vi "Load_Linnerud.vi"(8 "error in":errorcluster caption="entrée d'erreur") -> (0 "error out":errorcluster caption="sortie d'erreur", 3 "Tableau":string[][](array[string]))   [LabVIEW 2020]
doc: "Data Set Characteristics :\n\nNumber of Instances : 20\n\nNumber of Attributes : 3\n\nMissing Attribute Values : None\n\nThe Linnerud dataset is a multi-output regression dataset. It consists of three excercise (data) and three physiological (target) variables collected from twenty middle-aged men in a fitness club :\n\n - physiological - CSV containing 20 observations on 3 physiological variables : Weight, Waist and Pulse.\n\n - exercise - CSV containing 20 observations on 3 exercise variables : Chins, Situps and Jumps."
uses:
  Load_Linnerud.lvclass
panel:
  out "Load_Linnerud en sortie":refnum<class "Load_Linnerud.lvclass">
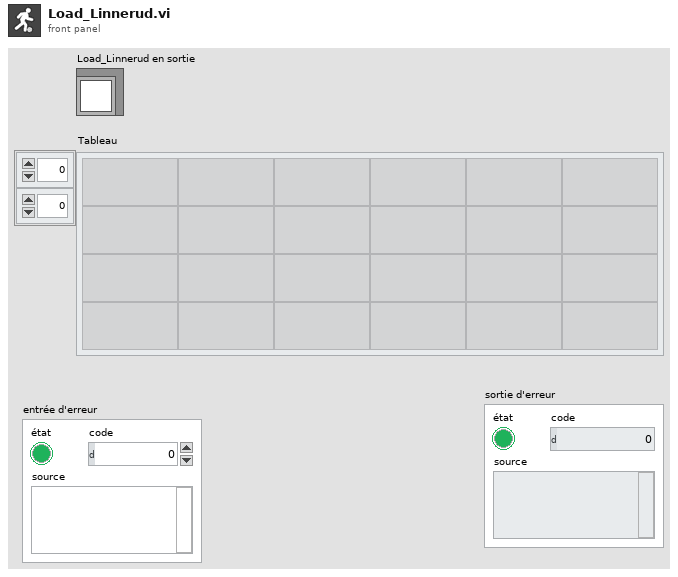
[diagram p1: front panel]
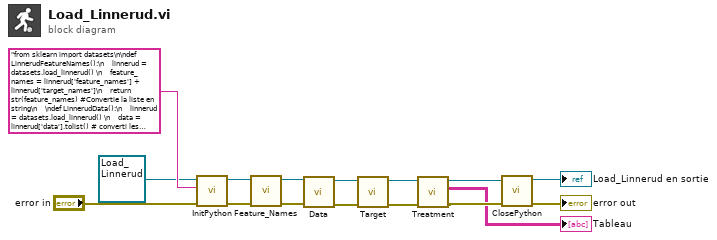
[diagram p0: block diagram]
diagram:
  n1 = call-dynamic "InitPython.vi"("error in (no error)"="error in", "Python Instruction"="from sklearn import datasets\n\ndef LinnerudFeatureNames():\n    linnerud = datasets.load_linnerud() \n    feature_names = linnerud['feature_names'] + linnerud['target_names']\n    return str(feature_names) #Convertie la liste en string\n    \ndef LinnerudData():\n    linnerud = datasets.load_linnerud() \n    data = linnerud['data'].tolist() # converti les datas en une liste\n    return str(data) #Convertie la liste en string\n\ndef LinnerudTarget():\n    linnerud = datasets.load_linnerud() \n    data_target = linnerud['target'].tolist() # converti les datas en une liste\n    return str(data_target) #Convertie la liste en string\n", "Scikit-learn en entrée"=refnum<class "Load_Linnerud.lvclass"> refnum ("Load_Linnerud.lvclass")) -> ("error out"=w11:errorcluster, "Scikit-learn en sortie"=w12:refnum<class "Load_Linnerud.lvclass">)  [unwired: 7 in]
  n2 = call-dynamic "Feature_Names.vi"("error in (no error)"=w11, "Load_Linnerud en entrée"=w12) -> ("error out"=w8:errorcluster, "Load_Linnerud en sortie"=w10:refnum<class "Load_Linnerud.lvclass">)  [unwired: 8 in]
  n3 = call-dynamic "Data.vi"("error in (no error)"=w8, "Load_Linnerud en entrée"=w10) -> ("error out"=w7:errorcluster, "Load_Linnerud en sortie"=w9:refnum<class "Load_Linnerud.lvclass">)  [unwired: 8 in]
  n4 = call-dynamic "Target.vi"("error in (no error)"=w7, "Load_Linnerud en entrée"=w9) -> ("error out"=w5:errorcluster, "Load_Linnerud en sortie"=w6:refnum<class "Load_Linnerud.lvclass">)  [unwired: 8 in]
  n5 = call-dynamic "Treatment.vi"("error in (no error)"=w5, "Load_Linnerud en entrée"=w6) -> ("error out"=w4:errorcluster, "Tableau"=→"Tableau":string[][], "Load_Linnerud en sortie"=w3:refnum<class "Load_Linnerud.lvclass">)  [unwired: 7 in]
  n6 = call-dynamic "ClosePython.vi"("error in (no error)"=w4, "Scikit-learn en entrée"=w3) -> ("error out"=→"error out":errorcluster, "Scikit-learn en sortie"=→"Load_Linnerud en sortie":refnum<class "Load_Linnerud.lvclass">)  [unwired: 8 in]
